vi "SR830 query XYR.vi"(0 "VISA resource name":refnum<visa-resource-name>, 11 "error in (no error)":errorcluster) -> (4 "VISA resource name out":refnum<visa-resource-name>, 6 "X":dbl, 8 "Y":dbl, 10 "R":dbl, 13 "Ch 1 display":dbl, 14 "Aux In 1":dbl, 15 "error out":errorcluster)   [LabVIEW 2017, in "SR830.lvlib"]
uses:
  SR830.lvlib
panel:
  out "read buffer":string
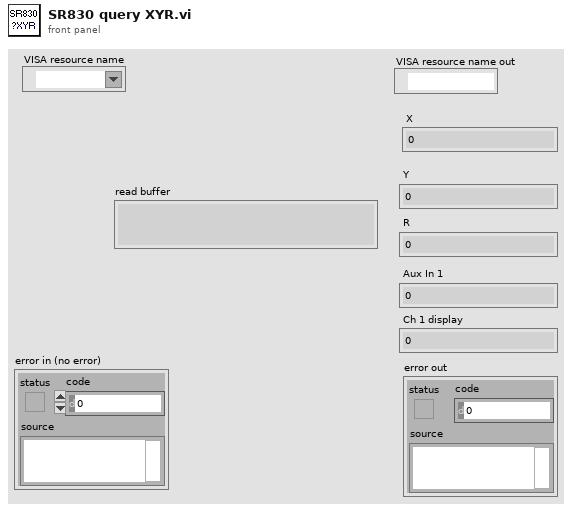
[diagram p1: front panel]
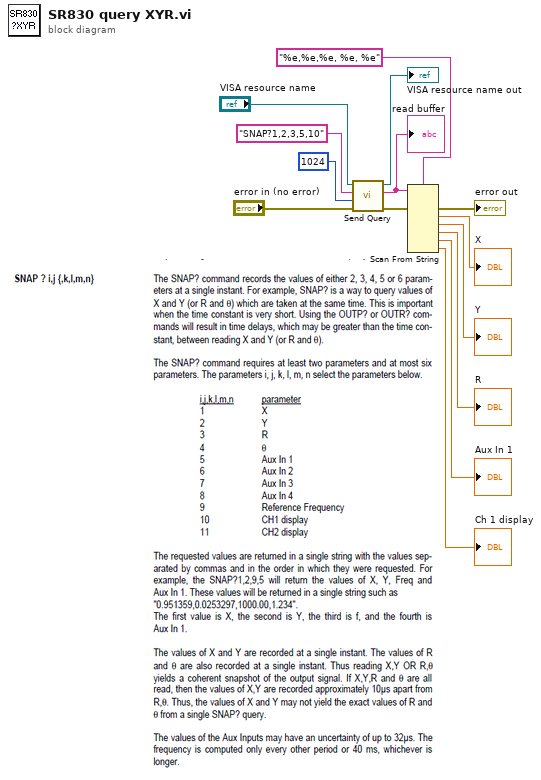
[diagram p0: block diagram]
diagram:
  n1 = call "Send Query.vi"("error in (no error)"="error in (no error)", "Bytes Count"=u32 1024 ("bytes to read (1000)"), "write buffer"="SNAP?1,2,3,5,10", "VISA resource name"="VISA resource name") -> ("error out"=w4:errorcluster, "read buffer"=w9:string, "VISA resource name out"=→"VISA resource name out":refnum<visa-resource-name>)  [unwired: 5 in]
  "read buffer" <- w9
  n2 = Scan From String(format string="%e,%e,%e, %e, %e", input string=w9, error in=w4) -> (error out=→"error out":errorcluster, output 1=→"X":dbl, output 2=→"Y":dbl, output 3=→"R":dbl, output 4=→"Aux In 1":dbl, output 5=→"Ch 1 display":dbl)  [unwired: 6 in, 2 out]
